vi "enumerateStaticDependencies.vi"(8 "error in (no error)":errorcluster, 11 "UI.Lockin":refnum<class "UI.Lockin.lvclass">) -> (0 "error out":errorcluster, 2 "Static Dependencies":refnum<class "Dependency.lvclass">[](array[class]), 3 "UI.Lockin out":refnum<class "UI.Lockin.lvclass">)   [LabVIEW 2019, in "UI.Lockin.lvclass"]
uses:
  UI.Lockin.lvclass
  <vilib>/JKI/JKI SMO/Dependency/Dependency.lvclass
  UI_Scope/UI.Lockin.Scope.lvclass
  C:/Program Files (x86)/National Instruments/LabVIEW 2019/user.lib/LevyLab/Instrument Framework/SMOs/Instrument UI/Instrument UI.lvclass
  UI_Generator_Config/UI.Lockin.Generator_Config.lvclass
  UI_DSP_Config/UI.Lockin.DSP_Config.lvclass
  UI_DAQ_config/UI.Lockin.DAQ_config.lvclass
  UI.Lockin.lvclass/UI.Lockin.ctl
  lockin/multichannel-lockin.lvclass
  C:/Program Files (x86)/National Instruments/LabVIEW 2019/user.lib/LevyLab/Instrument Framework/SMOs/Instrument/Instrument.lvclass
  <vilib>/Utility/VariantDataType/GetClusterInfo.vi
  <vilib>/Utility/VariantDataType/GetTypeInfo.vi
  <userlib>/LevyLab/Instrument Framework/SMOs/Instrument UI/Instrument UI.lvclass
  <vilib>/JKI/JKI SMO/SMO/SMO.lvclass
  C:/Program Files (x86)/National Instruments/LabVIEW 2019/vi.lib/JKI/JKI SMO/SMO.UI/SMO.UI.lvclass
  C:/Program Files (x86)/National Instruments/LabVIEW 2019/vi.lib/JKI/JKI SMO/SMO/SMO.lvclass
panel:
  # "For instructions on how to use the JKI State Machine Objects, examples and video tutorials, visit:\nhttp://jki.net/state-machine-objects/\n\nJKI State Machine Objects™\nhttp://jki.net/state-machine-objects/\nCopyright (C) 2005-2015, JKI <info@jki.net>\nALL RIGHTS RESERVED"
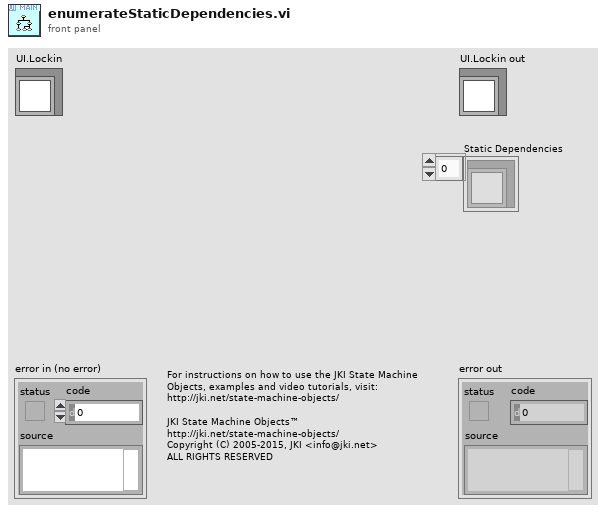
[diagram p1: front panel]
types:
  T1 = typedef "UI.Lockin.lvclass/SubUIs.ctl" = cluster{"UI_DAQ_cfg":refnum<class "UI.Lockin.DAQ_config.lvclass">, "UI_DSP_cfg":refnum<class "UI.Lockin.DSP_Config.lvclass">, "UI_Generator_cfg":refnum<class "UI.Lockin.Generator_Config.lvclass">, "UI_Scope":refnum<class "UI.Lockin.Scope.lvclass">}
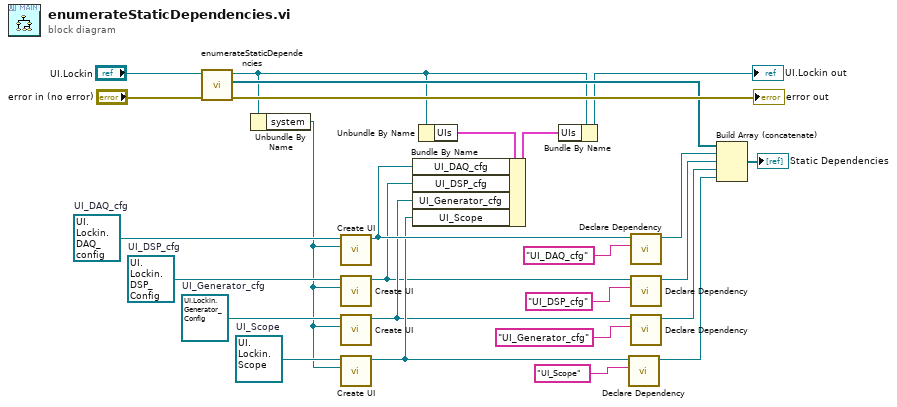
[diagram p0: block diagram]
diagram:
  w21 = refnum<class "UI.Lockin.DAQ_config.lvclass"> refnum  # UI_DAQ_cfg
  w20 = refnum<class "UI.Lockin.DSP_Config.lvclass"> refnum  # UI_DSP_cfg
  w19 = refnum<class "UI.Lockin.Generator_Config.lvclass"> refnum  # UI_Generator_cfg
  w18 = refnum<class "UI.Lockin.Scope.lvclass"> refnum  # UI_Scope
  n1 = call-parent "enumerateStaticDependencies.vi"("error in (no error)"="error in (no error)", "SMO"="UI.Lockin") -> ("error out"=→"error out":errorcluster, "Static Dependencies"=w22:refnum<class "Dependency.lvclass">[], "SMO out"=w15:refnum<class "UI.Lockin.lvclass">)  [unwired: 7 in]
  n2 = Unbundle By Name(w15) -> ("system"=w17:refnum<class "multichannel-lockin.lvclass">)
  n3 = call <userlib>:"Create UI.vi"("Instrument in"=w17, "Instrument UI"=w21) -> ("Instrument UI out"=w12:refnum<class "UI.Lockin.DAQ_config.lvclass">)  [unwired: 8 in, 1 out]
  n4 = call <userlib>:"Create UI.vi"("Instrument in"=w17, "Instrument UI"=w20) -> ("Instrument UI out"=w9:refnum<class "UI.Lockin.DSP_Config.lvclass">)  [unwired: 8 in, 1 out]
  n5 = call <userlib>:"Create UI.vi"("Instrument in"=w17, "Instrument UI"=w19) -> ("Instrument UI out"=w10:refnum<class "UI.Lockin.Generator_Config.lvclass">)  [unwired: 8 in, 1 out]
  n6 = call <userlib>:"Create UI.vi"("Instrument in"=w17, "Instrument UI"=w18) -> ("Instrument UI out"=w11:refnum<class "UI.Lockin.Scope.lvclass">)  [unwired: 8 in, 1 out]
  n7 = Unbundle By Name(w15) -> ("UIs"=w16:T1)
  n8 = Bundle By Name(cluster=w16, "UI_DAQ_cfg"=w12, "UI_DSP_cfg"=w9, "UI_Generator_cfg"=w10, "UI_Scope"=w11) -> (w13:T1)
  n9 = Bundle By Name(cluster=w15, "UIs"=w13) -> (→"UI.Lockin out":refnum<class "UI.Lockin.lvclass">)
  n10 = call <vilib>:"Declare Dependency.vi"("Name"="UI_Scope", "Type"=w11) -> ("Dependency out"=w1:refnum<class "Dependency.lvclass">)  [unwired: 8 in, 1 out]
  n11 = call <vilib>:"Declare Dependency.vi"("Name"="UI_DAQ_cfg", "Type"=w12) -> ("Dependency out"=w4:refnum<class "Dependency.lvclass">)  [unwired: 8 in, 1 out]
  n12 = call <vilib>:"Declare Dependency.vi"("Name"="UI_DSP_cfg", "Type"=w9) -> ("Dependency out"=w3:refnum<class "Dependency.lvclass">)  [unwired: 8 in, 1 out]
  n13 = call <vilib>:"Declare Dependency.vi"("Name"="UI_Generator_cfg", "Type"=w10) -> ("Dependency out"=w2:refnum<class "Dependency.lvclass">)  [unwired: 8 in, 1 out]
  n14 = Build Array (concatenate)(w22, w4, w3, w2, w1) -> (→"Static Dependencies":refnum<class "Dependency.lvclass">[])
